vi "LimitTests.vi"() -> ()   [LabVIEW 2014]
uses:
  <vilib>/Rock Robotics/SystemInterfaces/DIO/FPGA_DIOChannel.ctl
  <vilib>/Rock Robotics/SystemInterfaces/Typedef/FPGA_TypedefDigitalModule.ctl
  <vilib>/Rock Robotics/WPI/Switch/WPI_SwitchOpenLimit.vi
panel:
  out "Ejector Backward Initial Value":bool
  out "Ejector Forward Initial Value":bool
  out "Arms Open Initial Value":bool
  out "Elevator Bottom Initial Value":bool
  out "Elevator Top Initial Value":bool
  out "Ejector Backward Functional":bool
  out "Ejector Forward Functional":bool
  out "Arms Open Functional":bool
  out "Elevator Bottom Functional":bool
  out "Elevator Top Functional":bool
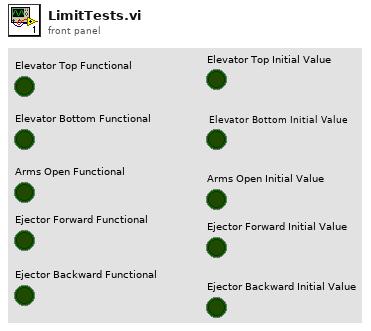
[diagram p1: front panel]
types:
  T1 = typedef "FPGA_DIOChannel.ctl" = enum8{"DIO 0", "DIO 1", "DIO 2", "DIO 3", "DIO 4", "DIO 5", "DIO 6", "DIO 7", "DIO 8", "DIO 9", "DIO MXP 0", "DIO MXP 1", "DIO MXP 2", "DIO MXP 3", "DIO MXP 4", "DIO MXP 5", "DIO MXP 6", "DIO MXP 7", "DIO MXP 8", "DIO MXP 9", "DIO MXP 10", "DIO MXP 11", "DIO MXP 12", "DIO MXP 13", "DIO MXP 14", "DIO MXP 15", "Invalid"}
  T2 = typedef "FPGA_TypedefDigitalModule.ctl" = enum16{"Controller 1"}
  T3 = typedef "WPI_SwitchDevRef.ctl" = cluster{"DevStatus":errorcluster, "DIO Channel":T1, "Controller":T2, "CntIndex":T4, "Normally Closed":bool}
  T4 = typedef "FPGA_CounterCtrSystemIndex.ctl" = enum8{"Ctr 0", "Ctr 1", "Ctr 2", "Ctr 3", "Ctr 4", "Ctr 5", "Ctr 6", "Ctr 7", "Invalid"}
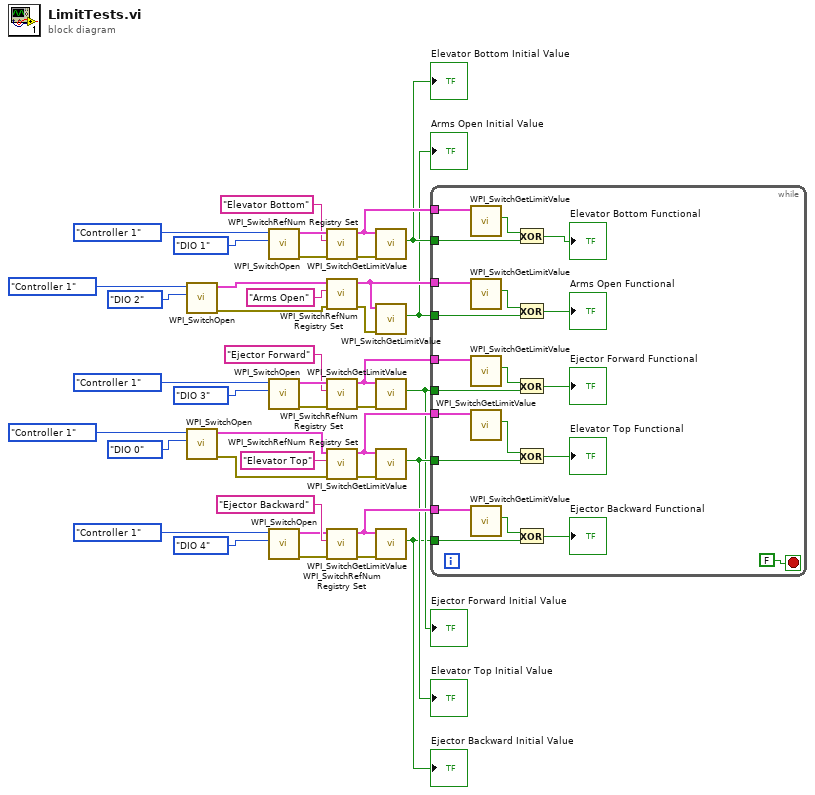
[diagram p0: block diagram]
diagram:
  n1 = call-poly <vilib>:"WPI_SwitchOpen.vi"("DIO Channel"=FPGA_DIOChannel."DIO 2", "Controller"=FPGA_TypedefDigitalModule."Controller 1") -> ("error out"=w28:errorcluster, "SwitchDevRef"=w29:T3)  [unwired: 8 in]
  n2 = call-poly <vilib>:"WPI_SwitchOpen.vi"("DIO Channel"=FPGA_DIOChannel."DIO 0", "Controller"=FPGA_TypedefDigitalModule."Controller 1") -> ("error out"=w38:errorcluster, "SwitchDevRef"=w37:T3)  [unwired: 8 in]
  n3 = call-poly <vilib>:"WPI_SwitchOpen.vi"("DIO Channel"=FPGA_DIOChannel."DIO 1", "Controller"=FPGA_TypedefDigitalModule."Controller 1") -> ("error out"=w33:errorcluster, "SwitchDevRef"=w32:T3)  [unwired: 8 in]
  n4 = call-poly <vilib>:"WPI_SwitchOpen.vi"("DIO Channel"=FPGA_DIOChannel."DIO 3", "Controller"=FPGA_TypedefDigitalModule."Controller 1") -> ("error out"=w23:errorcluster, "SwitchDevRef"=w22:T3)  [unwired: 8 in]
  n5 = call-poly <vilib>:"WPI_SwitchOpen.vi"("DIO Channel"=FPGA_DIOChannel."DIO 4", "Controller"=FPGA_TypedefDigitalModule."Controller 1") -> ("error out"=w18:errorcluster, "SwitchDevRef"=w19:T3)  [unwired: 8 in]
  n6 = call <vilib>:"WPI_SwitchRefNum Registry Set.vi"("error in (no error)"=w33, "refnum name"="Elevator Bottom", "SwitchDevRef"=w32) -> ("error out"=w11:errorcluster, "SwitchDevRef"=w8:T3)  [unwired: 7 in]
  n7 = call <vilib>:"WPI_SwitchRefNum Registry Set.vi"("error in (no error)"=w28, "refnum name"="Arms Open", "SwitchDevRef"=w29) -> ("error out"=w14:errorcluster, "SwitchDevRef"=w9:T3)  [unwired: 7 in]
  n8 = call <vilib>:"WPI_SwitchRefNum Registry Set.vi"("error in (no error)"=w23, "refnum name"="Ejector Forward", "SwitchDevRef"=w22) -> ("error out"=w13:errorcluster, "SwitchDevRef"=w10:T3)  [unwired: 7 in]
  n9 = call <vilib>:"WPI_SwitchRefNum Registry Set.vi"("error in (no error)"=w38, "refnum name"="Elevator Top", "SwitchDevRef"=w37) -> ("error out"=w15:errorcluster, "SwitchDevRef"=w7:T3)  [unwired: 7 in]
  n10 = call <vilib>:"WPI_SwitchRefNum Registry Set.vi"("error in (no error)"=w18, "refnum name"="Ejector Backward", "SwitchDevRef"=w19) -> ("error out"=w12:errorcluster, "SwitchDevRef"=w6:T3)  [unwired: 7 in]
  n11 = call <vilib>:"WPI_SwitchGetLimitValue.vi"("error in (no error)"=w11, "SwitchDevRef"=w8) -> ("Switch Pressed"=w5:bool)  [unwired: 7 in, 2 out]
  "Elevator Bottom Initial Value" <- w5
  n12 = call <vilib>:"WPI_SwitchGetLimitValue.vi"("error in (no error)"=w14, "SwitchDevRef"=w9) -> ("Switch Pressed"=w4:bool)  [unwired: 7 in, 2 out]
  "Arms Open Initial Value" <- w4
  n13 = call <vilib>:"WPI_SwitchGetLimitValue.vi"("error in (no error)"=w13, "SwitchDevRef"=w10) -> ("Switch Pressed"=w2:bool)  [unwired: 7 in, 2 out]
  "Ejector Forward Initial Value" <- w2
  n14 = call <vilib>:"WPI_SwitchGetLimitValue.vi"("error in (no error)"=w15, "SwitchDevRef"=w7) -> ("Switch Pressed"=w3:bool)  [unwired: 7 in, 2 out]
  "Elevator Top Initial Value" <- w3
  n15 = call <vilib>:"WPI_SwitchGetLimitValue.vi"("error in (no error)"=w12, "SwitchDevRef"=w6) -> ("Switch Pressed"=w1:bool)  [unwired: 7 in, 2 out]
  "Ejector Backward Initial Value" <- w1
  n16 = while {
    tunnel: w3 -> [w49]
    tunnel: w5 -> [w51]
    tunnel: w4 -> [w53]
    tunnel: w2 -> [w55]
    tunnel: w1 -> [w47]
    tunnel: w10 -> [w61]
    tunnel: w9 -> [w60]
    tunnel: w8 -> [w59]
    tunnel: w7 -> [w58]
    tunnel: w6 -> [w57]
    stop <- FALSE stop-if-true
    n17 = call <vilib>:"WPI_SwitchGetLimitValue.vi"("SwitchDevRef"=w59) -> ("Switch Pressed"=w52:bool)  [unwired: 8 in, 2 out]
    n18 = call <vilib>:"WPI_SwitchGetLimitValue.vi"("SwitchDevRef"=w60) -> ("Switch Pressed"=w54:bool)  [unwired: 8 in, 2 out]
    n19 = call <vilib>:"WPI_SwitchGetLimitValue.vi"("SwitchDevRef"=w61) -> ("Switch Pressed"=w56:bool)  [unwired: 8 in, 2 out]
    n20 = call <vilib>:"WPI_SwitchGetLimitValue.vi"("SwitchDevRef"=w58) -> ("Switch Pressed"=w50:bool)  [unwired: 8 in, 2 out]
    n21 = call <vilib>:"WPI_SwitchGetLimitValue.vi"("SwitchDevRef"=w57) -> ("Switch Pressed"=w48:bool)  [unwired: 8 in, 2 out]
    n22 = Exclusive Or(1:w51, 2:w52) -> (0:→"Elevator Bottom Functional":bool)
    n23 = Exclusive Or(1:w53, 2:w54) -> (0:→"Arms Open Functional":bool)
    n24 = Exclusive Or(1:w55, 2:w56) -> (0:→"Ejector Forward Functional":bool)
    n25 = Exclusive Or(1:w49, 2:w50) -> (0:→"Elevator Top Functional":bool)
    n26 = Exclusive Or(1:w47, 2:w48) -> (0:→"Ejector Backward Functional":bool)
  }
